vi "alignment.vi"() -> ()   [LabVIEW 2021]
uses:
  <vilib>/Instr/_visa.llb/VISA Configure Serial Port (Instr).vi
panel:
  in  "duration half cycle":dbl=0.5
  out "Device name":string
  in  "VISA resource name":refnum<visa-resource-name>="COM7"
  in  "stop":bool
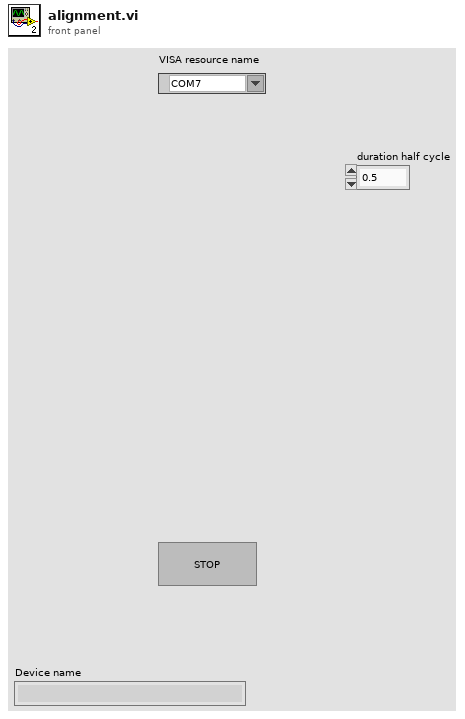
[diagram p1: front panel]
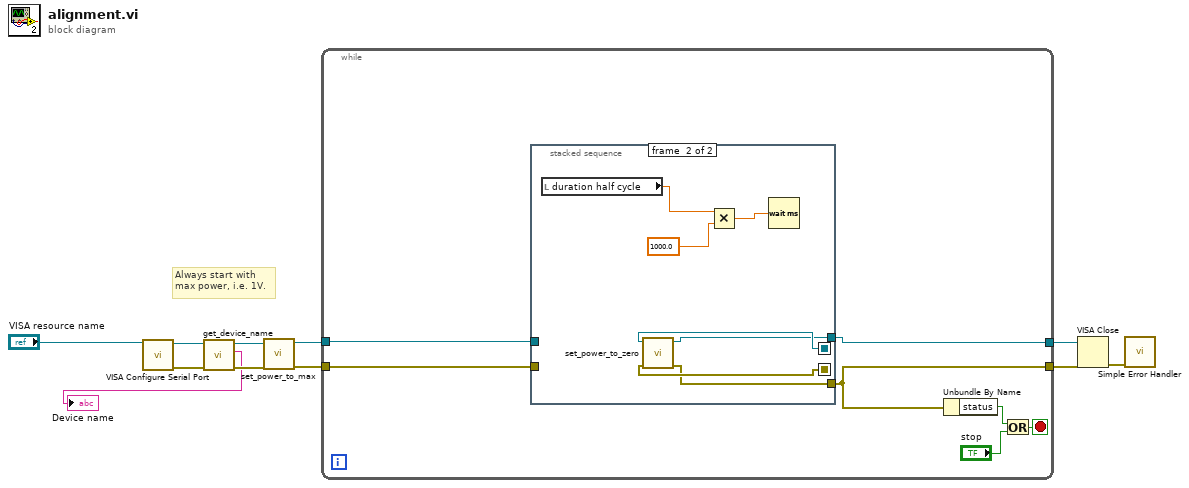
[diagram p0: block diagram]
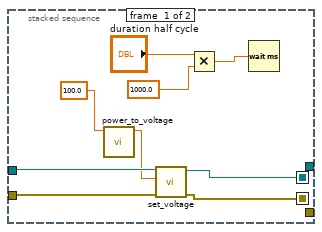
[diagram p2: hidden frame]
diagram:
  # "Always start with\nmax power, i.e. 1V."
  n1 = call-poly "VISA Configure Serial Port"("VISA resource name"="VISA resource name") -> ("VISA resource name out"=w2:refnum<visa-resource-name>, "error out"=w3:errorcluster)  [unwired: 9 in, 4 out]
  n2 = call "get_device_name.vi"("error in"=w3, "VISA resource name in"=w2) -> ("error out"=w4:errorcluster, "Device name"=→"Device name":string, "VISA resource name out"=w5:refnum<visa-resource-name>)  [unwired: 7 in]
  n3 = call "set_power_to_max.vi"("error in"=w4, "VISA resource name"=w5) -> ("error out"=w10:errorcluster, "VISA resource name out"=w11:refnum<visa-resource-name>)  [unwired: 8 in]
  n4 = while {
    tunnel: w11 -> [w17]
    tunnel: w10 -> [w16]
    tunnel: [w12] -> w7
    tunnel: [w13] -> w6
    stop <- w18 stop-if-true
    n5 = stacked-sequence {
      seq-local: [w20 _] -> [_ w30]
      seq-local: [w19 _] -> [_ w31]
      tunnel: w17 -> [w26 _]
      tunnel: w16 -> [w27 _]
      tunnel: [_ w29] -> w13
      tunnel: [_ w28] -> w12
      frame #0 {
        n6 = call "power_to_voltage.vi"("Power"=100.0) -> ("Voltage"=w25:dbl)  [unwired: 10 in]
        n7 = call "set_voltage.vi"("error in"=w27, "voltage"=w25, "VISA resource name"=w26) -> ("error out"=w19:errorcluster, "VISA resource name out"=w20:refnum<visa-resource-name>)  [unwired: 6 in, 1 out]
        n8 = Multiply(x="duration half cycle", y=1000.0) -> (x*y=w23:dbl)
        n9 = Wait (ms)(milliseconds to wait=w23) -> ()  [unwired: 1 out]
      }
      frame #1 {
        n10 = local read "duration half cycle"() -> (w32:dbl)
        n11 = call "set_power_to_zero.vi"("error in"=w31, "VISA resource name"=w30) -> ("error out"=w28:errorcluster, "VISA resource name out"=w29:refnum<visa-resource-name>)  [unwired: 8 in]
        n12 = Multiply(x=w32, y=1000.0) -> (x*y=w34:dbl)
        n13 = Wait (ms)(milliseconds to wait=w34) -> ()  [unwired: 1 out]
      }
    }
    n14 = Unbundle By Name(w12) -> ("status"=w15:bool)
    n15 = Or(x=w15, y="stop") -> (x .or. y?=w18:bool)
  }
  n16 = VISA Close(VISA resource name=w6, error in (no error)=w7) -> (error out=w8:errorcluster)
  n17 = call <vilib>:"Simple Error Handler.vi"("error in (no error)"=w8) -> ()  [unwired: 1 in, 8 out]
